vi "lab5_euler.vi"(0 "a":dbl, 1 "b":dbl, 2 "Array":dbl[][](array[numeric]), 3 "шаг по времени":dbl, 4 "конец по времени":dbl) -> (5 "Array out":dbl[](array[numeric]))   [LabVIEW 2018]
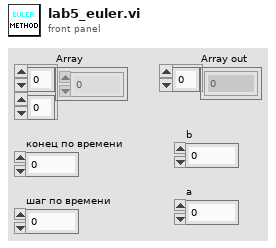
[diagram p1: front panel]
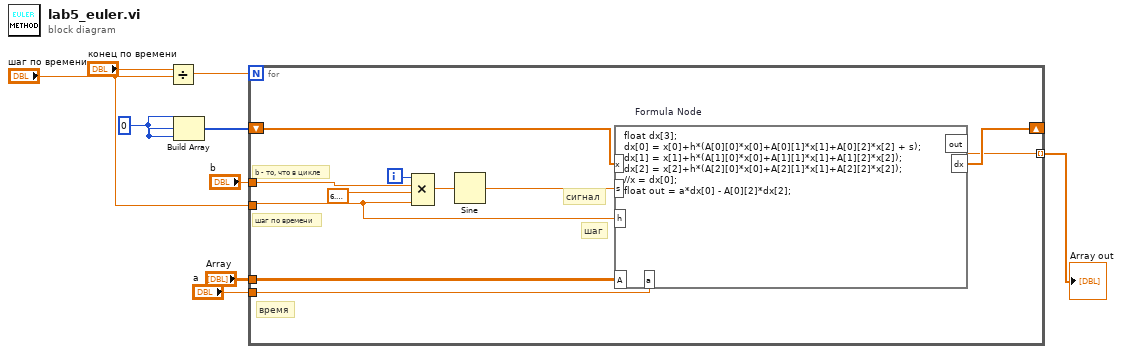
[diagram p0: block diagram]
diagram:
  w3 = 0
  n1 = Divide(x="конец по времени", y="шаг по времени") -> (x/y=w4:dbl)
  n2 = Build Array(w3, w3, w3) -> (w2:i32[])
  n3 = for {
    N: w4 -> [_]
    tunnel: "b" -> [w19]
    tunnel: "шаг по времени" -> [w15]
    tunnel: [w14] -> w7 mode=indexing
    shift-right: [w16] -> _
    shift-left: w2 -> [w17]
    tunnel: "a" -> [w12]
    tunnel: "Array" -> [w11]
    i -> [w13]
    # "шаг по времени"
    # "b - то, что в цикле"
    # "время"
    # "шаг"
    # "сигнал"
    n4 = Compound Arithmetic op=MULTIPLY(6.283185307179586, w19, w13, w15) -> (w18:dbl)
    n5 = Sine(x=w18) -> (sin(x)=w10:dbl)
    n6 = formula code="float dx[3];\ndx[0] = x[0]+h*(A[0][0]*x[0]+A[0][1]*x[1]+A[0][2]*x[2] + s);\ndx[1] = x[1]+h*(A[1][0]*x[0]+A[1][1]*x[1]+A[1][2]*x[2]);\ndx[2] = x[2]+h*(A[2][0]*x[0]+A[2][1]*x[1]+A[2][2]*x[2]);\n//x = dx[0];\nfloat out = a*dx[0] - A[0][2]*dx[2];"("x"=w17, "s"=w10, "h"=w15, "A"=w11, "a"=w12) -> ("dx"=w16:dbl[], "out"=w14:dbl)
  }
  "Array out" <- w7
